vi "Color Table.vi"(7 "_Table":refnum<vi>, 11 "Colors":u32[](array[colorbox])) -> ()   [LabVIEW 2015, in "ECS-Host.lvlib"]
uses:
  <vilib>/Utility/miscctls.llb/LVRowAndColumnTypeDef.ctl
  ECS-Host.lvlib
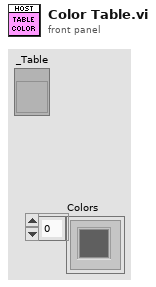
[diagram p1: front panel]
types:
  T1 = typedef "LVRowAndColumnTypeDef.ctl" = cluster{"Row":i32, "Column":i32}
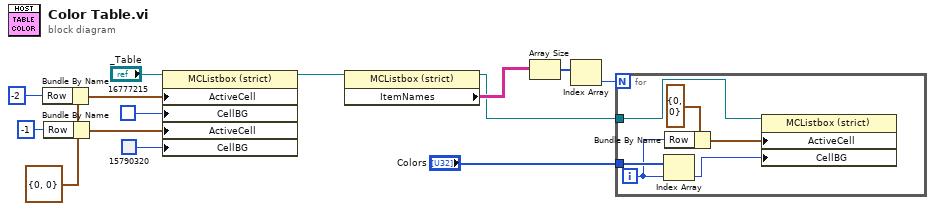
[diagram p0: block diagram]
diagram:
  w11 = T1 {"Row"=0, "Column"=0} ("Active Cell:Active Cell")
  n1 = Bundle By Name(cluster=w11, "Row"=-2) -> (w9:T1)
  n2 = Bundle By Name(cluster=w11, "Row"=-1) -> (w13:T1)
  n3 = property on="Property Node" class="MCListbox (strict)"(reference="_Table", "ActiveCell"=w9, "CellBG"=u32 16777215, "ActiveCell"=w13, "CellBG"=u32 15790320) -> (reference out=w2:refnum<vi>)  [unwired: 1 in, 1 out]
  n4 = property on="Property Node" class="MCListbox (strict)"(reference=w2) -> (reference out=w1:refnum<vi>, "ItemNames"=w3:string[][])  [unwired: 1 in, 1 out]
  n5 = Array Size(array=w3) -> (size(s)=w7:i32[])
  n6 = Index Array(array=w7) -> (element=w6:i32)  [unwired: 1 in]
  n7 = for {
    N: w6 -> [_]
    tunnel: "Colors" -> [w20]
    tunnel: w1 -> [w17]
    i -> [w16]
    n8 = Index Array(array=w20, index=w16) -> (element=w15:u32)
    n9 = Bundle By Name(cluster=T1 {"Row"=0, "Column"=0} ("Active Cell:Active Cell"), "Row"=w16) -> (w18:T1)
    n10 = property on="Property Node" class="MCListbox (strict)"(reference=w17, "ActiveCell"=w18, "CellBG"=w15) -> ()  [unwired: 1 in, 2 out]
  }
